vi "ExerciceReservoir.vi"() -> ()   [LabVIEW 2018]
uses:
  ExerciceReservoir/Control 4.ctl
  ExerciceReservoir/Control 3.ctl
  ExerciceReservoir/Control 2.ctl
panel:
  in  "?":bool
  in  "Consigne":T1 max=1000 scale=0.0..1000.0
  in  "Débit":T2=1 min=1 max=10 scale=1.0..10.0
  out "Réservoir":T3 scale=0.0..1100.0
  # "[l/s]"
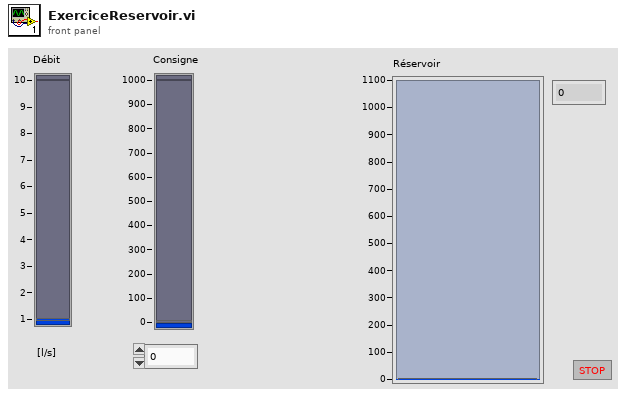
[diagram p1: front panel]
types:
  T1 = typedef "Control 2.ctl" = u16
  T2 = typedef "Control 3.ctl" = u8
  T3 = typedef "Control 4.ctl" = u16
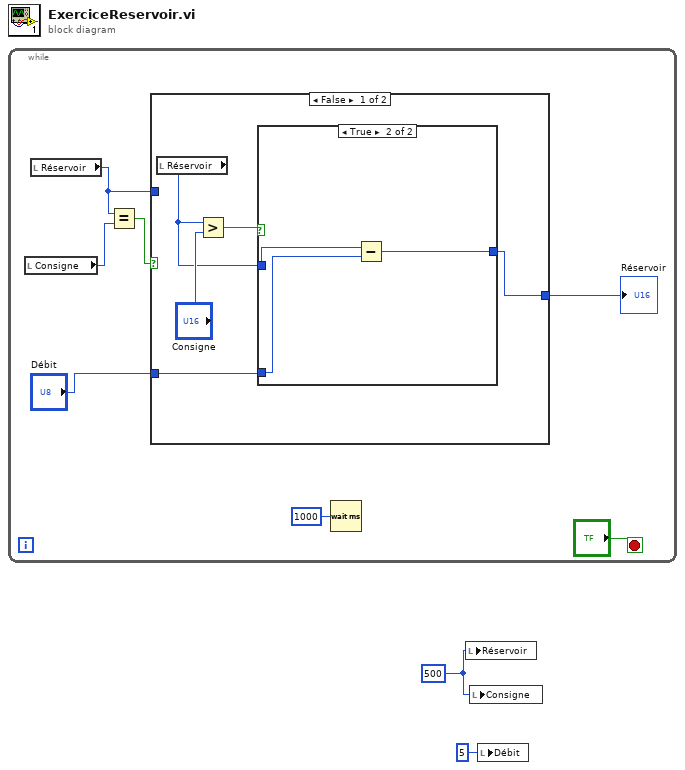
[diagram p0: block diagram]
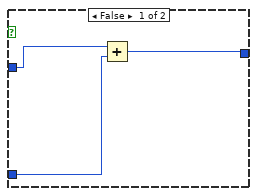
[diagram p2: hidden frame]
diagram:
  w2 = T3 500 ("Réservoir")
  n1 = while {
    stop <- "?" stop-if-true
    n2 = local read "Consigne"() -> (w7:T1)
    n3 = local read "Réservoir"() -> (w4:T3)
    n4 = Equal?(x=w4, y=w7) -> (x = y?=w5:bool)
    n5 = case shown="False" w5 {
      tunnel: [w11 w21] -> w6
      tunnel: w4 -> [_ w21]
      tunnel: "Débit" -> [w10 _]
      frame False {
        n6 = local read "Réservoir"() -> (w12:T3)
        n7 = Greater?(x=w12, y="Consigne") -> (0:w13:bool)
        n8 = case shown="True" w13 {
          tunnel: [w16 w20] -> w11
          tunnel: w12 -> [w17 w19]
          tunnel: w10 -> [w15 w18]
          frame False {
            n9 = Add(x=w17, y=w15) -> (x+y=w16:T3)
          }
          frame True {
            n10 = Subtract(x=w19, y=w18) -> (x-y=w20:T3)
          }
        }
      }
      frame True {
      }
    }
    "Réservoir" <- w6
    n11 = Wait (ms)(milliseconds to wait=u32 1000) -> ()  [unwired: 1 out]
  }
  n12 = local write "Réservoir"(w2) -> ()
  n13 = local write "Consigne"(w2) -> ()
  n14 = local write "Débit"(T2 5 ("Débit")) -> ()
